vi "Single action pushbutton latching program.vi"() -> ()   [LabVIEW 2013]
panel:
  out "Boolean":bool
  in  "Single action pushbutton":bool
  in  "Stop Program":bool
  out "Output LED":bool
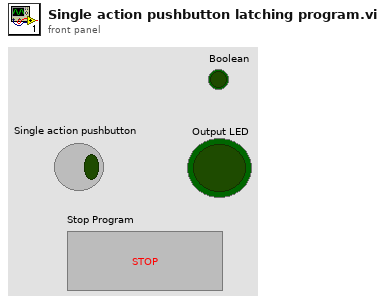
[diagram p1: front panel]
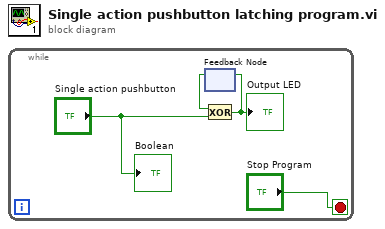
[diagram p0: block diagram]
diagram:
  n1 = while {
    stop <- "Stop Program" stop-if-true
    n2 = feedback #1() -> (w3:bool)  [unwired: 1 in]
    n3 = Exclusive Or(1:"Single action pushbutton", 2:w3) -> (0:w2:bool)
    "Output LED" <- w2
    n4 = feedback-in #1(w2) -> ()
    "Boolean" <- "Single action pushbutton"
  }
